vi "Bind To Name.vi"(8 "error in (no error)":errorcluster, 10 "Type":refnum<class>, 11 "Default Serialization Binder in":refnum<class "Default Serialization Binder.lvclass">) -> (0 "error out":errorcluster, 2 "Type Name":string, 3 "Default Serialization Binder out":refnum<class "Default Serialization Binder.lvclass">)   [LabVIEW 2017, in "Default Serialization Binder.lvclass"]
doc: "Controls the binding of a type to a serialized object."
uses:
  Default Serialization Binder.lvclass
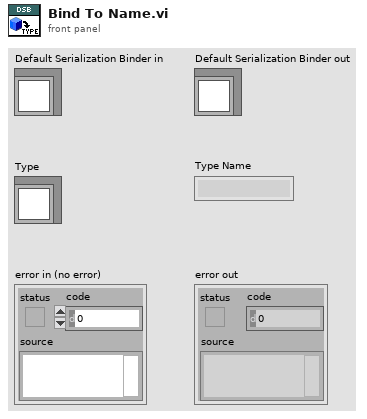
[diagram p1: front panel]
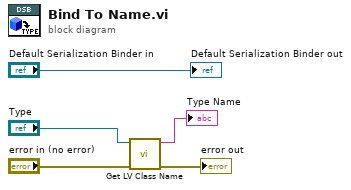
[diagram p0: block diagram]
diagram:
  n1 = call <vilib>:"Get LV Class Name.vi"("error in (no error)"="error in (no error)", "object"="Type") -> ("error out"=→"error out":errorcluster, "class name"=→"Type Name":string)  [unwired: 8 in]
  "Default Serialization Binder out" <- "Default Serialization Binder in"
